vi "SiosIfmSetToZero.vi"(0 "Channel1":bool, 1 "Channel2":bool, 2 "Channel3":bool, 3 "Channel4":bool, 4 "deviceNumber":i32) -> (5 "success":i32)   [LabVIEW 2009]
uses:
  siosifm.dll
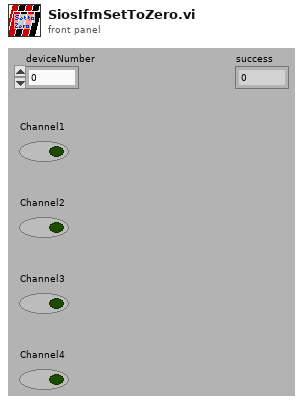
[diagram p1: front panel]
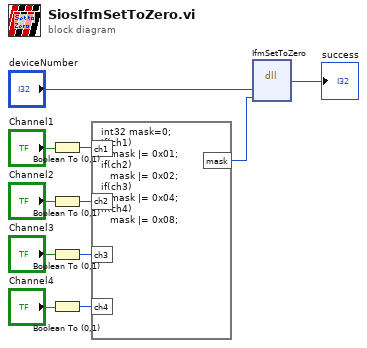
[diagram p0: block diagram]
diagram:
  n1 = Boolean To (0,1)(Boolean="Channel1") -> (0, 1=w7:i16)
  n2 = Boolean To (0,1)(Boolean="Channel2") -> (0, 1=w6:i16)
  n3 = Boolean To (0,1)(Boolean="Channel3") -> (0, 1=w5:i16)
  n4 = Boolean To (0,1)(Boolean="Channel4") -> (0, 1=w4:i16)
  n5 = formula code="int32 mask=0;\nif(ch1)\n   mask |= 0x01;\nif(ch2)\n   mask |= 0x02;\nif(ch3)\n   mask |= 0x04;\nif(ch4)\n   mask |= 0x08;"("ch1"=w7, "ch2"=w6, "ch3"=w5, "ch4"=w4) -> ("mask"=w2:i32)
  n6 = dll-call lib="D:/Support/Labview/RE-10/SIOS_IfmDLL/siosifm.dll" fn="IfmSetToZero"("deviceNumber"="deviceNumber", "channelMask"=w2) -> ("return type"=→"success":i32)  [unwired: 5 in, 2 out]
